vi "DC Bus Test_TS_BB.vi"(1 "Board Selector":T1, 5 "error in (no error)":errorcluster) -> (0 "INV A (10V)":dbl, 2 "INV B (10V)":dbl, 6 "INV A (0V)":dbl, 7 "INV B (0V)":dbl)   [LabVIEW 2022 SP3]
uses:
  Serial Board Com/Board Select.ctl
  Serial Board Com/ADCSelector BB.ctl
  HMP4000 Communication/HMP4040_ChannelControl.ctl
  Serial Board Com/ADCSelector GB.ctl
panel:
  out "error out":errorcluster
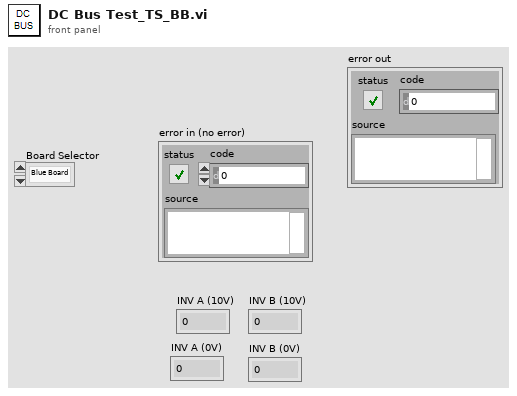
[diagram p1: front panel]
types:
  T1 = typedef "Board Select.ctl" = enum16{"Blue Board", "Green Board"}
  T2 = typedef "ADCSelector GB.ctl" = enum16{"INVA_ISENSE_U", "INVA_ISENSE_V", "INVA_ISENSE_W", "INVA_UDC", "INVA_TEMP", "HB_ISENSE", "AUX_ISENSE_U", "AUX_ISENSE_V", "AUX_ISENSE_W", "VLINE_AB", "VLINE_BC", "VLINE_CA", "REF_1P5V", "VSENSE_POS_24V", "VSENSE_POS_5V", "VSENSE_NEG_15V", "TEST_POINT", "INVB_ISENSE_U", "INVB_ISENSE_V", "INVB_ISENSE_W", "INVB_UDC", "INVB_TEMP", "HB_TEMP", "AUXA_TEMP", "AUXB_TEMP", "AUXC_TEMP", "VOUT_AB", "VOUT_BC", "VOUT_CA", "REF_2P5V", "VSENSE_POS_15V", "VSENSE_POS_3P3V", "NET_ANALYZER"}
  T3 = typedef "HMP4040_ChannelControl.ctl" = cluster{"CH1 Voltage":dbl, "CH1 Current":dbl, "CH1 Output":bool, "CH2 Voltage":dbl, "CH2 Current":dbl, "CH2 Output":bool, "CH3 Voltage":dbl, "CH3 Current":dbl, "CH3 Output":bool, "CH4 Voltage":dbl, "CH4 Current":dbl, "CH4 Output":bool, "Master Output":bool}
  T4 = typedef "ADCSelector BB.ctl" = enum16{"INVA_ISENSE_U", "INVA_ISENSE_V", "INVA_ISENSE_W", "INVA_UDC", "INVA_TEMP", "HB_TEMP", "AUXB_TEMP", "VLINE_AB", "VLINE_BC", "VLINE_CA", "VSENSE_POS_24V", "VSENSE_POS_5V", "VSENSE_NEG_15V", "INVB_ISENSE_U", "INV_B_ISENSEV", "INVB_ISENSE_W", "INVB_UDC", "INVB_TEMP", "AUXA_TEMP", "AUXC_TEMP", "VOUT_AB", "VOUT_BC", "VOUT_CA", "VSENSE_POS_15V", "VSENSE_POS_3P3V", "TEST_POINT"}
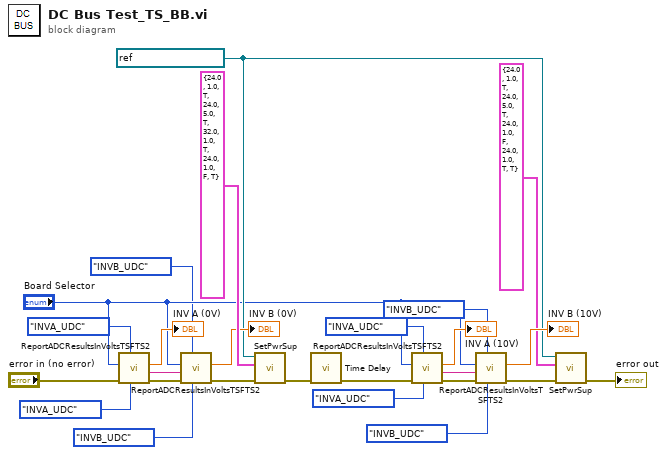
[diagram p0: block diagram]
diagram:
  w11 = refnum<visa-resource-name> "HMP4040_FTS2" ("Power Supply")
  n1 = call "ReportADCResultsInVoltsTSFTS2.vi"("Blue Board Enum"=ADCSelector_BB."INVA_UDC", "Green Board Enum"=ADCSelector_GB."INVA_UDC", "error in (no error)"="error in (no error)", "Board Selector"="Board Selector") -> ("error out"=w24:errorcluster, "Message OUT"=w22:string, "Result"=→"INV A (0V)":dbl)  [unwired: 4 in, 1 out]
  n2 = call "ReportADCResultsInVoltsTSFTS2.vi"("Blue Board Enum"=ADCSelector_BB."INVB_UDC", "Green Board Enum"=ADCSelector_GB."INVB_UDC", "error in (no error)"=w24, "Message IN"=w22, "Board Selector"="Board Selector") -> ("error out"=w21:errorcluster, "Result"=→"INV B (0V)":dbl)  [unwired: 3 in, 2 out]
  n3 = call "SetPwrSup.vi"("error in (no error)"=w21, "HMP4040 Channel Settings"=T3 {"CH1 Voltage"=24.0, "CH1 Current"=1.0, "CH1 Output"=TRUE, "CH2 Voltage"=24.0, "CH2 Current"=5.0, "CH2 Output"=TRUE, "CH3 Voltage"=32.0, "CH3 Current"=1.0, "CH3 Output"=TRUE, "CH4 Voltage"=24.0, "CH4 Current"=1.0, "CH4 Output"=FALSE, "Master Output"=TRUE}, "HMP4040 IN"=w11) -> ("error out"=w25:errorcluster)  [unwired: 7 in, 1 out]
  n4 = call "Time Delay"("error in (no error)"=w25) -> ("error out"=w16:errorcluster)  [unwired: 10 in]
  n5 = call "ReportADCResultsInVoltsTSFTS2.vi"("Blue Board Enum"=ADCSelector_BB."INVA_UDC", "Green Board Enum"=ADCSelector_GB."INVA_UDC", "error in (no error)"=w16, "Board Selector"="Board Selector") -> ("error out"=w19:errorcluster, "Message OUT"=w17:string, "Result"=→"INV A (10V)":dbl)  [unwired: 4 in, 1 out]
  n6 = call "ReportADCResultsInVoltsTSFTS2.vi"("Blue Board Enum"=ADCSelector_BB."INVB_UDC", "Green Board Enum"=ADCSelector_GB."INVB_UDC", "error in (no error)"=w19, "Message IN"=w17, "Board Selector"="Board Selector") -> ("error out"=w13:errorcluster, "Result"=→"INV B (10V)":dbl)  [unwired: 3 in, 2 out]
  n7 = call "SetPwrSup.vi"("error in (no error)"=w13, "HMP4040 Channel Settings"=T3 {"CH1 Voltage"=24.0, "CH1 Current"=1.0, "CH1 Output"=TRUE, "CH2 Voltage"=24.0, "CH2 Current"=5.0, "CH2 Output"=TRUE, "CH3 Voltage"=24.0, "CH3 Current"=1.0, "CH3 Output"=FALSE, "CH4 Voltage"=24.0, "CH4 Current"=1.0, "CH4 Output"=TRUE, "Master Output"=TRUE}, "HMP4040 IN"=w11) -> ("error out"=→"error out":errorcluster)  [unwired: 7 in, 1 out]
